vi "Read ADC Type.vi"(8 "Error In":errorcluster, 11 "Adc Convertor In":refnum<class "Adc Convertor.lvclass">) -> (0 "Error Out":errorcluster, 2 "Adc Type":T1={"Channels"="", "Range"=0.0, "Resolution"=2.0, "Sampling Rate"=0.0} {"Resolution" min=2.0 max=16.0}, 3 "Adc Convertor Out":refnum<class "Adc Convertor.lvclass">)   [LabVIEW 2021, in "Adc Convertor.lvclass"]
uses:
  Adc Convertor.lvclass
  Controls/ADC Type.ctl
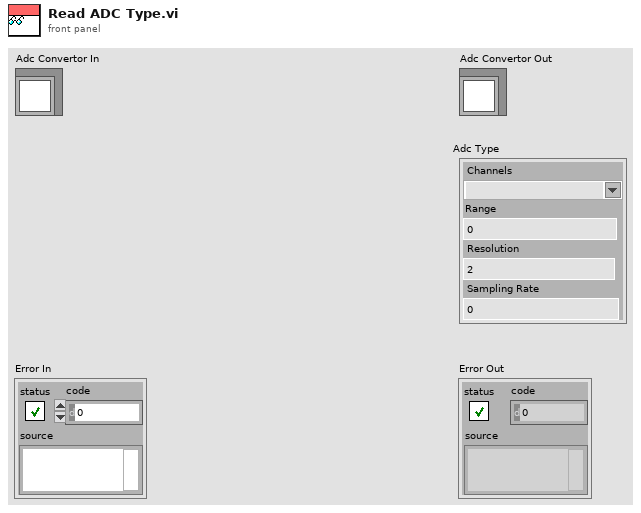
[diagram p1: front panel]
types:
  T1 = typedef "ADC Type.ctl" = cluster{"Channels":string, "Range":dbl, "Resolution":dbl, "Sampling Rate":dbl}
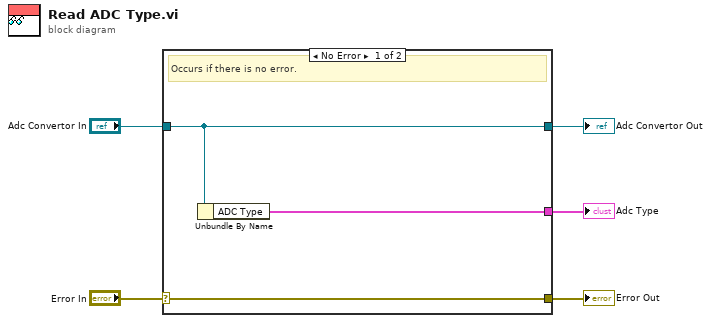
[diagram p0: block diagram]
diagram:
  n1 = case shown="No Error" "Error In" {
    selector: "Error In" -> [w8 w9]
    tunnel: [w8 w9] -> w4
    tunnel: [w7 w10] -> w2
    tunnel: "Adc Convertor In" -> [w7 w10]
    tunnel: [w6 _] -> w1
    frame No Error {
      # "Occurs if there is no error."
      n2 = Unbundle By Name(w7) -> ("ADC Type"=w6:T1)
    }
    frame Error {
      # "Occurs if there is any error."
    }
  }
  "Error Out" <- w4
  "Adc Convertor Out" <- w2
  "Adc Type" <- w1
